vi "Power interface Check if Magna and determin type.vi"(0 "VISA Refnum in":refnum<visa-resource-name>, 11 "error in (no error)":errorcluster) -> (8 "PSU type":T1, 13 "Found PSU":bool, 15 "error out":errorcluster)   [LabVIEW 2011]
uses:
  PCP interface/PSU Type.ctl
  <vilib>/Instr/_visa.llb/VISA Configure Serial Port (Instr).vi
  <vilib>/regexp/Match Regular Expression.xnode
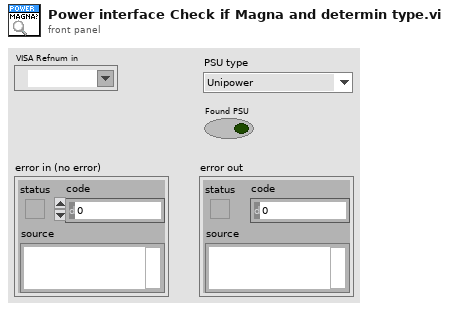
[diagram p1: front panel]
types:
  T1 = typedef "PSU Type.ctl" = enum16{"Unipower", "Magna 8.3A", "Magna 12A", "None"}
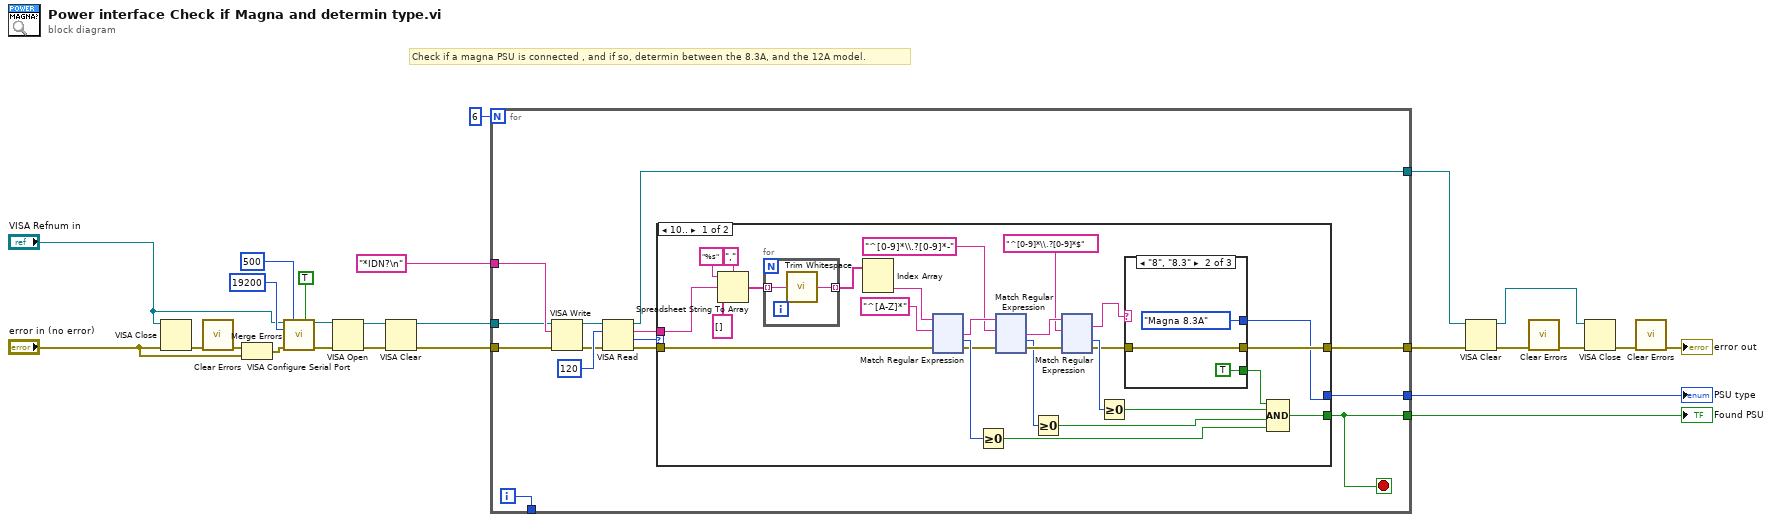
[diagram p0: block diagram]
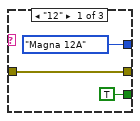
[diagram p2: hidden frame]
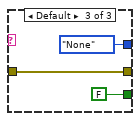
[diagram p3: hidden frame]
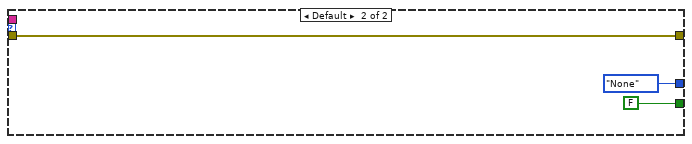
[diagram p4: hidden frame]
diagram:
  # "Check if a magna PSU is connected , and if so, determin between the 8.3A, and the 12A model."
  n1 = VISA Close(VISA resource name="VISA Refnum in", error in (no error)="error in (no error)") -> (error out=w15:errorcluster)
  n2 = call <vilib>:"Clear Errors.vi"("error in (no error)"=w15) -> ("error out"=w16:errorcluster)  [unwired: 6 in]
  n3 = Merge Errors(w16, "error in (no error)") -> (w17:errorcluster)
  n4 = call-poly "VISA Configure Serial Port"("VISA resource name"="VISA Refnum in", "timeout (10sec)"=u32 500, "Enable Termination\nChar (T)"=TRUE ("Enable Termination\nChar (T)"), "baud rate (9600)"=u32 19200, "error in (no error)"=w17) -> ("VISA resource name out"=w11:refnum<visa-resource-name>, "error out"=w12:errorcluster)  [unwired: 9 in]
  n5 = VISA Open(error in (no error)=w12, VISA resource name=w11) -> (VISA resource name=w14:refnum<visa-resource-name>, error out=w13:errorcluster)  [unwired: 3 in]
  n6 = VISA Clear(VISA resource name=w14, error in (no error)=w13) -> (VISA resource name out=w21:refnum<visa-resource-name>, error out=w20:errorcluster)
  n7 = for {
    N: 6 -> [_]
    tunnel: [w39] -> w25
    tunnel: [w27] -> w24
    tunnel: "*IDN?\n" -> [w32]
    tunnel: w21 -> [w31]
    tunnel: w20 -> [w30]
    tunnel: [w29] -> w9
    tunnel: [w28] -> w8
    tunnel: [w26] -> _
    i -> [w26]
    stop <- w27 stop-if-true
    n8 = VISA Write(VISA resource name=w31, write buffer=w32, error in (no error)=w30) -> (VISA resource name out=w34:refnum<visa-resource-name>, error out=w33:errorcluster)  [unwired: 1 out]
    n9 = VISA Read(VISA resource name=w34, byte count=u32 120, error in (no error)=w33) -> (VISA resource name out=w28:refnum<visa-resource-name>, read buffer=w38:string, return count=w36:u32, error out=w37:errorcluster)
    n10 = case shown="10.." w36 {
      tunnel: w37 -> [w59 w413]
      tunnel: [w43 w413] -> w29
      tunnel: w38 -> [w61 _]
      tunnel: [w42 FALSE] -> w27
      tunnel: [w41 PSU_Type."None" ("PSU type")] -> w39
      frame 10.. {
        n11 = Spreadsheet String To Array(delimiter (Tab)=",", format string="%s", spreadsheet string=w61, array type (2D Dbl)=string[] []) -> (array=w63:string[])
        n12 = for {
          tunnel: w63 -> [w410] mode=indexing
          tunnel: [w409] -> w62 mode=indexing
          n13 = call <vilib>:"Trim Whitespace.vi"("string"=w410) -> ("trimmed string"=w409:string)  [unwired: 1 in]
        }
        n14 = Index Array(array=w62) -> (element #2=w60:string)  [unwired: 2 in, 1 out]
        n15 = xnode "Match Regular Expression"("input string"=w60, "regular expression"="^[A-Z]*" ("element"), "error in"=w59) -> ("after match"=w56:string, "offset past match"=w57:i32, "error out"=w52:errorcluster)  [unwired: 3 in, 2 out]
        n16 = Greater Or Equal To 0?(x=w57) -> (x >= 0?=w45:bool)
        n17 = xnode "Match Regular Expression"("input string"=w56, "regular expression"="^[0-9]*\\.?[0-9]*-" ("element"), "error in"=w52) -> ("after match"=w55:string, "offset past match"=w50:i32, "error out"=w51:errorcluster)  [unwired: 3 in, 2 out]
        n18 = Greater Or Equal To 0?(x=w50) -> (x >= 0?=w46:bool)
        n19 = xnode "Match Regular Expression"("input string"=w55, "regular expression"="^[0-9]*\\.?[0-9]*$" ("element"), "error in"=w51) -> ("whole match"=w40:string, "offset past match"=w49:i32, "error out"=w48:errorcluster)  [unwired: 3 in, 2 out]
        n20 = Greater Or Equal To 0?(x=w49) -> (x >= 0?=w47:bool)
        n21 = case shown="\"8\", \"8.3\"" w40 {
          tunnel: w48 -> [w68 w71 w74]
          tunnel: [TRUE TRUE FALSE] -> w44
          tunnel: [w68 w71 w74] -> w43
          tunnel: [PSU_Type."Magna 12A" ("PSU type") PSU_Type."Magna 8.3A" ("PSU type") PSU_Type."None" ("PSU type")] -> w41
          frame "12" {
          }
          frame "8", "8.3" {
          }
          frame Default {
          }
        }
        n22 = Compound Arithmetic op=AND(w44, w47, w46, w45) -> (w42:bool)
      }
      frame Default {
      }
    }
  }
  "PSU type" <- w25
  "Found PSU" <- w24
  n23 = VISA Clear(VISA resource name=w8, error in (no error)=w9) -> (VISA resource name out=w4:refnum<visa-resource-name>, error out=w3:errorcluster)
  n24 = call <vilib>:"Clear Errors.vi"("error in (no error)"=w3) -> ("error out"=w2:errorcluster)  [unwired: 6 in]
  n25 = VISA Close(VISA resource name=w4, error in (no error)=w2) -> (error out=w5:errorcluster)
  n26 = call <vilib>:"Clear Errors.vi"("error in (no error)"=w5) -> ("error out"=→"error out":errorcluster)  [unwired: 6 in]
